vi "停止整机测试(子VI).vi"() -> (0 "error out":T1={"status"=FALSE, "代码"=4, "source"=""} caption="错误输出" {"代码" items=["执行成功"=1, "执行失败，但不知道原因"=2, "命令请求条件错误"=3, "通讯超时"=4, "系统繁忙不能执行"=5, "系统故障"=6, "没有数据"=100]})   [LabVIEW 2016, in "MB SLAVE.lvlib"]
uses:
  MB SLAVE.lvlib
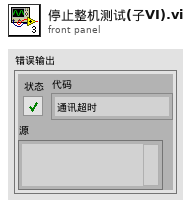
[diagram p1: front panel]
types:
  T1 = cluster{"status":bool, "代码":u16, "source":string}
  T2 = cluster{"命令":string, cluster{"starting address":u16, "holding register value":u16}}
  T3 = cluster{"命令":string, "测量模式":enum16{"水样测量", "标样核查", "零点核查", "跨度核查", "空白测试", "加标回收", "平行样", "校零", "校标"}, "CODMn量程切换":enum32{"H", "L", "AUTO"}}
  T4 = typedef "启动参数.ctl" = cluster{"氨氮":bool, "总磷":bool, "总氮":bool, "多参数":bool, "CODmn":bool, "CODCr":bool, "超标留样":bool}
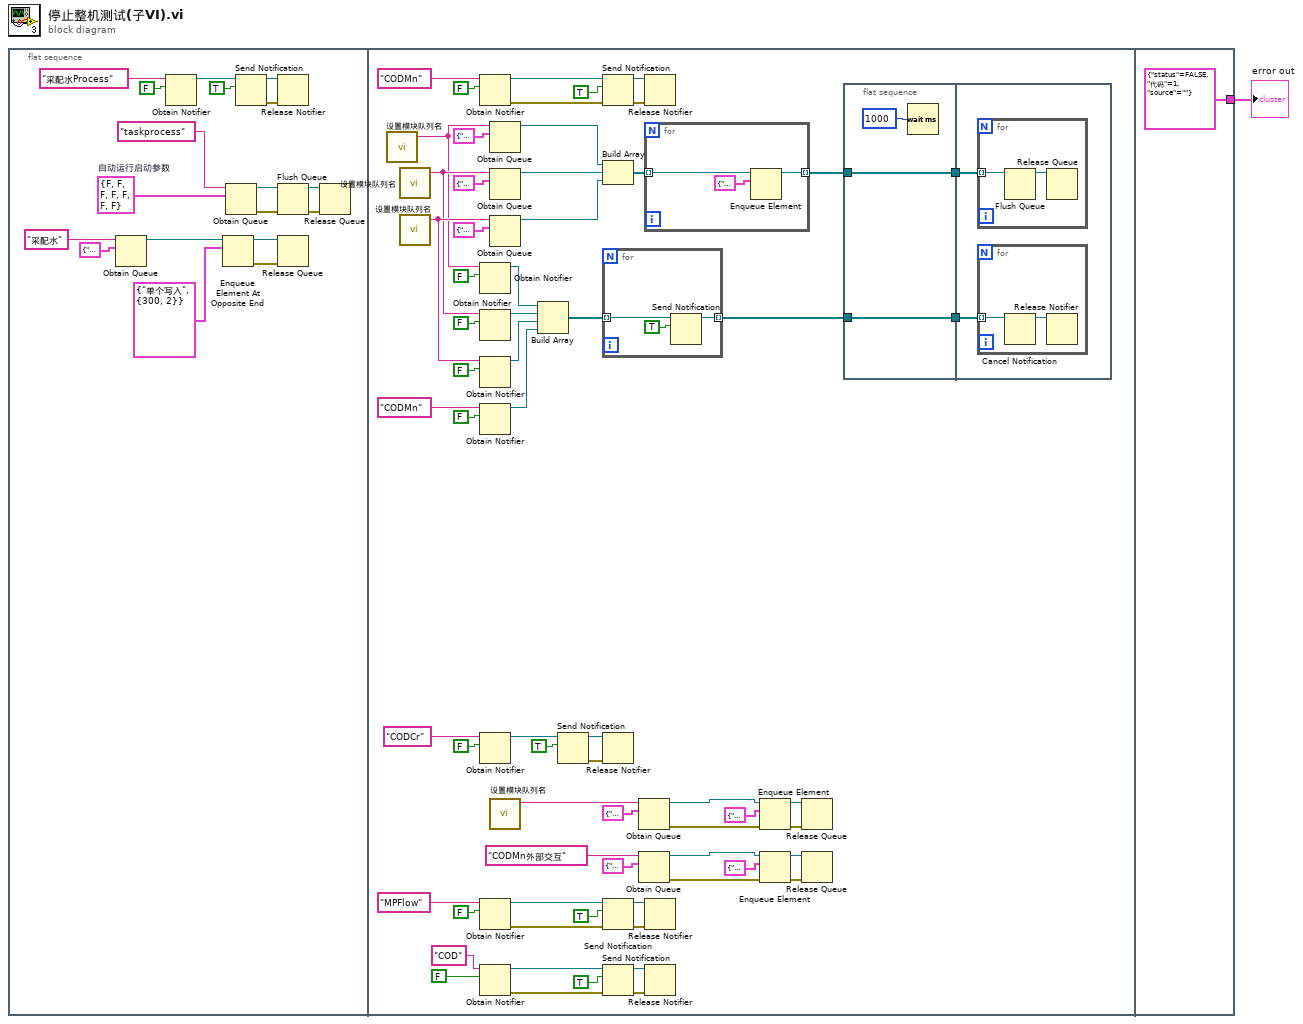
[diagram p0: block diagram]
diagram:
  n1 = flat-sequence {
    tunnel: [T1 {"status"=FALSE, "代码"=1, "source"=""} ("error out")] -> w1
    frame #0 {
      w2 = T4 {"氨氮"=FALSE, "总磷"=FALSE, "总氮"=FALSE, "多参数"=FALSE, "CODmn"=FALSE, "CODCr"=FALSE, "超标留样"=FALSE}  # 自动运行启动参数
      n2 = Obtain Queue(name (unnamed)="采配水" ("名称（未命名）"), element data type=cluster{"命令":string, "数据":variant} {"命令"="", "数据"=variant}) -> (queue out=w17:refnum<queue>)  [unwired: 3 in, 2 out]
      n3 = Obtain Notifier(name (unnamed)="采配水Process" ("名称（未命名）"), notification data type=FALSE) -> (notifier out=w19:refnum<notifier>)  [unwired: 2 in, 2 out]
      n4 = Enqueue Element At Opposite End(queue=w17, element=T2 {"命令"="单个写入", {"starting address"=300, "holding register value"=2}} ("元素")) -> (queue out=w11:refnum<queue>, error out=w10:errorcluster)  [unwired: 2 in, 1 out]
      n5 = Obtain Queue(name (unnamed)="taskprocess" ("名称（未命名）"), element data type=w2) -> (queue out=w6:refnum<queue>, error out=w5:errorcluster)  [unwired: 3 in, 1 out]
      n6 = Send Notification(notification=TRUE ("通知"), notifier=w19) -> (notifier out=w9:refnum<notifier>, error out=w8:errorcluster)  [unwired: 1 in]
      n7 = Release Notifier(notifier=w9, error in (no error)=w8) -> ()  [unwired: 1 in, 3 out]
      n8 = Flush Queue(queue=w6, error in (no error)=w5) -> (queue out=w3:refnum<queue>, error out=w4:errorcluster)  [unwired: 1 out]
      n9 = Release Queue(queue=w11, error in (no error)=w10) -> ()  [unwired: 1 in, 3 out]
      n10 = Release Queue(queue=w3, error in (no error)=w4) -> ()  [unwired: 1 in, 3 out]
    }
    frame #1 {
      n11 = call "设置模块队列名.vi"() -> ("Msg"=w20:string)  [unwired: 5 in]
      n12 = call "设置模块队列名.vi"() -> ("Msg"=w32:string)  [unwired: 5 in]
      n13 = call "设置模块队列名.vi"() -> ("Msg"=w35:string)  [unwired: 5 in]
      n14 = Obtain Notifier(name (unnamed)="CODMn" ("名称（未命名）"), notification data type=FALSE) -> (notifier out=w81:refnum<notifier>, error out=w58:errorcluster)  [unwired: 2 in, 1 out]
      n15 = Obtain Notifier(name (unnamed)=w20, notification data type=FALSE) -> (notifier out=w38:refnum<notifier>)  [unwired: 2 in, 2 out]
      n16 = Obtain Notifier(name (unnamed)=w32, notification data type=FALSE) -> (notifier out=w39:refnum<notifier>)  [unwired: 2 in, 2 out]
      n17 = Obtain Notifier(name (unnamed)=w35, notification data type=FALSE) -> (notifier out=w40:refnum<notifier>)  [unwired: 2 in, 2 out]
      n18 = Obtain Notifier(name (unnamed)="CODMn" ("名称（未命名）"), notification data type=FALSE) -> (notifier out=w41:refnum<notifier>)  [unwired: 2 in, 2 out]
      n19 = Obtain Notifier(name (unnamed)="CODCr" ("名称（未命名）"), notification data type=FALSE) -> (notifier out=w75:refnum<notifier>)  [unwired: 2 in, 2 out]
      n20 = Obtain Notifier(name (unnamed)="MPFlow" ("名称（未命名）"), notification data type=FALSE) -> (notifier out=w77:refnum<notifier>, error out=w76:errorcluster)  [unwired: 2 in, 1 out]
      n21 = Obtain Notifier(name (unnamed)="COD" ("名称（未命名）"), notification data type=FALSE) -> (notifier out=w62:refnum<notifier>, error out=w63:errorcluster)  [unwired: 2 in, 1 out]
      n22 = Obtain Queue(name (unnamed)=w20, element data type=cluster{"命令":string, "data":variant} {"命令"="", "data"=variant}) -> (queue out=w42:refnum<queue>)  [unwired: 3 in, 2 out]
      n23 = Obtain Queue(name (unnamed)=w32, element data type=cluster{"命令":string, "data":variant} {"命令"="", "data"=variant}) -> (queue out=w43:refnum<queue>)  [unwired: 3 in, 2 out]
      n24 = Obtain Queue(name (unnamed)=w35, element data type=cluster{"命令":string, "data":variant} {"命令"="", "data"=variant}) -> (queue out=w44:refnum<queue>)  [unwired: 3 in, 2 out]
      n25 = call "设置模块队列名.vi"() -> ("Msg"=w23:string)  [unwired: 11 in]
      n26 = Build Array(w38, w39, w40, w41) -> (w46:refnum<notifier>[])
      n27 = Send Notification(notification=TRUE ("通知"), notifier=w75) -> (notifier out=w69:refnum<notifier>, error out=w68:errorcluster)  [unwired: 1 in]
      n28 = Send Notification(notification=TRUE ("通知"), notifier=w81, error in (no error)=w58) -> (notifier out=w71:refnum<notifier>, error out=w70:errorcluster)
      n29 = Build Array(w42, w43, w44) -> (w45:refnum<queue>[])
      n30 = for {
        tunnel: w46 -> [w96] mode=indexing
        tunnel: [w94] -> w47 mode=indexing
        n31 = Send Notification(notification=TRUE ("通知"), notifier=w96) -> (notifier out=w94:refnum<notifier>)  [unwired: 1 in, 1 out]
      }
      n32 = Release Notifier(notifier=w69, error in (no error)=w68) -> ()  [unwired: 1 in, 3 out]
      n33 = Send Notification(notification=TRUE ("通知"), notifier=w77, error in (no error)=w76) -> (notifier out=w67:refnum<notifier>, error out=w66:errorcluster)
      n34 = Send Notification(notification=TRUE ("通知"), notifier=w62, error in (no error)=w63) -> (notifier out=w64:refnum<notifier>, error out=w65:errorcluster)
      n35 = Obtain Queue(name (unnamed)=w23, element data type=cluster{"命令":string, "data":variant} {"命令"="", "data"=variant}) -> (queue out=w24:refnum<queue>, error out=w25:errorcluster)  [unwired: 3 in, 1 out]
      n36 = Obtain Queue(name (unnamed)="CODMn外部交互" ("名称（未命名）"), element data type=T3 {"命令"="启动命令", "测量模式"=enum."水样测量", "CODMn量程切换"=enum."AUTO"} ("元素")) -> (queue out=w53:refnum<queue>, error out=w52:errorcluster)  [unwired: 3 in, 1 out]
      n37 = Release Notifier(notifier=w71, error in (no error)=w70) -> ()  [unwired: 1 in, 3 out]
      n38 = for {
        tunnel: w45 -> [w98] mode=indexing
        tunnel: [w97] -> w48 mode=indexing
        n39 = Enqueue Element(queue=w98, element=cluster{"命令":string, "data":variant} {"命令"="启动", "data"=variant(cluster{"站号":u16, "控制命令":u16[]} {"站号"=1, "控制命令"=[2816]})} ("启动命令")) -> (queue out=w97:refnum<queue>)  [unwired: 2 in, 2 out]
      }
      n40 = Release Notifier(notifier=w67, error in (no error)=w66) -> ()  [unwired: 1 in, 3 out]
      n41 = Release Notifier(notifier=w64, error in (no error)=w65) -> ()  [unwired: 1 in, 3 out]
      n42 = Enqueue Element(queue=w24, element=cluster{"命令":string, "data":variant} {"命令"="启动", "data"=variant(cluster{"站号":u16, "控制命令":u16[]} {"站号"=21, "控制命令"=[2816]})} ("启动命令"), error in (no error)=w25) -> (queue out=w26:refnum<queue>, error out=w27:errorcluster)  [unwired: 1 in, 1 out]
      n43 = Enqueue Element(queue=w53, element=T3 {"命令"="停止命令", "测量模式"=enum."水样测量", "CODMn量程切换"=enum."H"} ("元素"), error in (no error)=w52) -> (queue out=w55:refnum<queue>, error out=w54:errorcluster)  [unwired: 1 in, 1 out]
      n44 = Release Queue(queue=w26, error in (no error)=w27) -> ()  [unwired: 1 in, 3 out]
      n45 = Release Queue(queue=w55, error in (no error)=w54) -> ()  [unwired: 1 in, 3 out]
      n46 = flat-sequence {
        tunnel: w48 -> [w86]
        tunnel: w47 -> [w87]
        tunnel: [w87] -> w50
        tunnel: [w86] -> w49
        tunnel: w50 -> [w89]
        tunnel: w49 -> [w88]
        frame #0 {
          n47 = Wait (ms)(milliseconds to wait=u32 1000 ("等待时间（毫秒）")) -> ()  [unwired: 1 out]
        }
        frame #1 {
          n48 = for {
            tunnel: w88 -> [w91] mode=indexing
            n49 = Flush Queue(queue=w91) -> (queue out=w90:refnum<queue>)  [unwired: 1 in, 2 out]
            n50 = Release Queue(queue=w90) -> ()  [unwired: 2 in, 3 out]
          }
          n51 = for {
            tunnel: w89 -> [w93] mode=indexing
            n52 = Cancel Notification(0:w93) -> (8:w92:refnum<notifier>)  [unwired: 1 in, 2 out]
            n53 = Release Notifier(notifier=w92) -> ()  [unwired: 2 in, 3 out]
          }
        }
      }
    }
    frame #2 {
    }
  }
  "error out" <- w1
